vi "Get position.vi"(8 "error in (no error)":errorcluster, 11 "Dummy Motor in":refnum<class "Dummy Motor.lvclass">) -> (0 "error out":errorcluster, 2 "Position (rev)":dbl, 3 "Dummy Motor out":refnum<class "Dummy Motor.lvclass">)   [LabVIEW 2015, in "Dummy Motor.lvclass"]
uses:
  Dummy Motor.lvclass
  Dummy Motor.lvclass/Dummy Motor.ctl
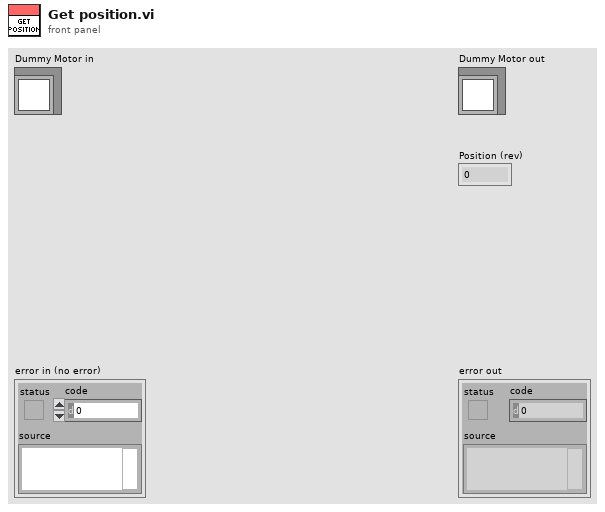
[diagram p1: front panel]
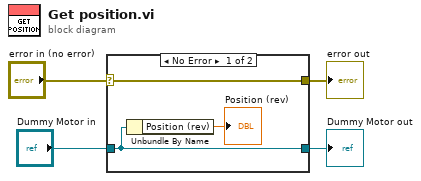
[diagram p0: block diagram]
diagram:
  n1 = case shown="No Error" "error in (no error)" {
    selector: "error in (no error)" -> [w7 w9]
    tunnel: [w7 w9] -> w3
    tunnel: "Dummy Motor in" -> [w5 w8]
    tunnel: [w5 w8] -> w1
    frame No Error {
      n2 = Unbundle By Name(w5) -> ("Position (rev)"=→"Position (rev)":dbl)
    }
    frame Error {
    }
  }
  "error out" <- w3
  "Dummy Motor out" <- w1
